vi "BotPose Correction.vi"(9 "Pos In":cluster{"x":dbl, "y":dbl}={"x"=13.014915967536774, "y"=9.532980345268305}, 10 "Robot Velocities In":T3={"X Velocity"=-6.0927338461737115e-19, "Y Velocity"=3.330663501205842e-16, "Rotational \nVelocity"=-0.0823974609375}) -> (0 "BotPose":cluster{"Numeric":dbl, "Numeric":dbl}, 1 "Bordeaux Pos":cluster{dbl, dbl}, 2 "Robot Velocities Out":T3={"X Velocity"=-6.0927338461737115e-19, "Y Velocity"=3.330663501205842e-16, "Rotational \nVelocity"=-0.0823974609375})   [LabVIEW 2025]
uses:
  swerve-template/Type Definitions/Data/Robot Velocities.ctl
  <vilib>/Rock Robotics/Network Tables/NT Read Numeric Array.vi
  <vilib>/addons/control/pid/pid.llb/PID (DBL).vi
  <vilib>/addons/control/pid/NI_PID_pid.lvlib
panel:
  in  "PID gains":T1={"proportional gain (Kc)"=2.5, "integral time (Ti, min)"=0.0, "derivative time (Td, min)"=0.0} {"derivative time (Td, min)" format="%.3f"; "integral time (Ti, min)" format="%.3f"; "proportional gain (Kc)" format="%.3f"}
  in  "output range":cluster{"output high":dbl, "output low":dbl}={"output high"=4.0, "output low"=-4.0} {"output low" format="%.2f"; "output high" format="%.2f"}
  out "Error":cluster{dbl, dbl}(graph)={-6.0927338461737115e-19, -1.21152228156357}
  out "Velocities OUT":T2(graph)={"X Velocity"=-6.0927338461737115e-19, "Y Velocity"=3.330663501205842e-16, "Rotational \nVelocity"=-0.0823974609375}
  out "Tag IDs":dbl(graph)=18.0
  out "Correction":cluster{dbl, dbl}(graph)={-6.0927338461737115e-19, -1.21152228156357}
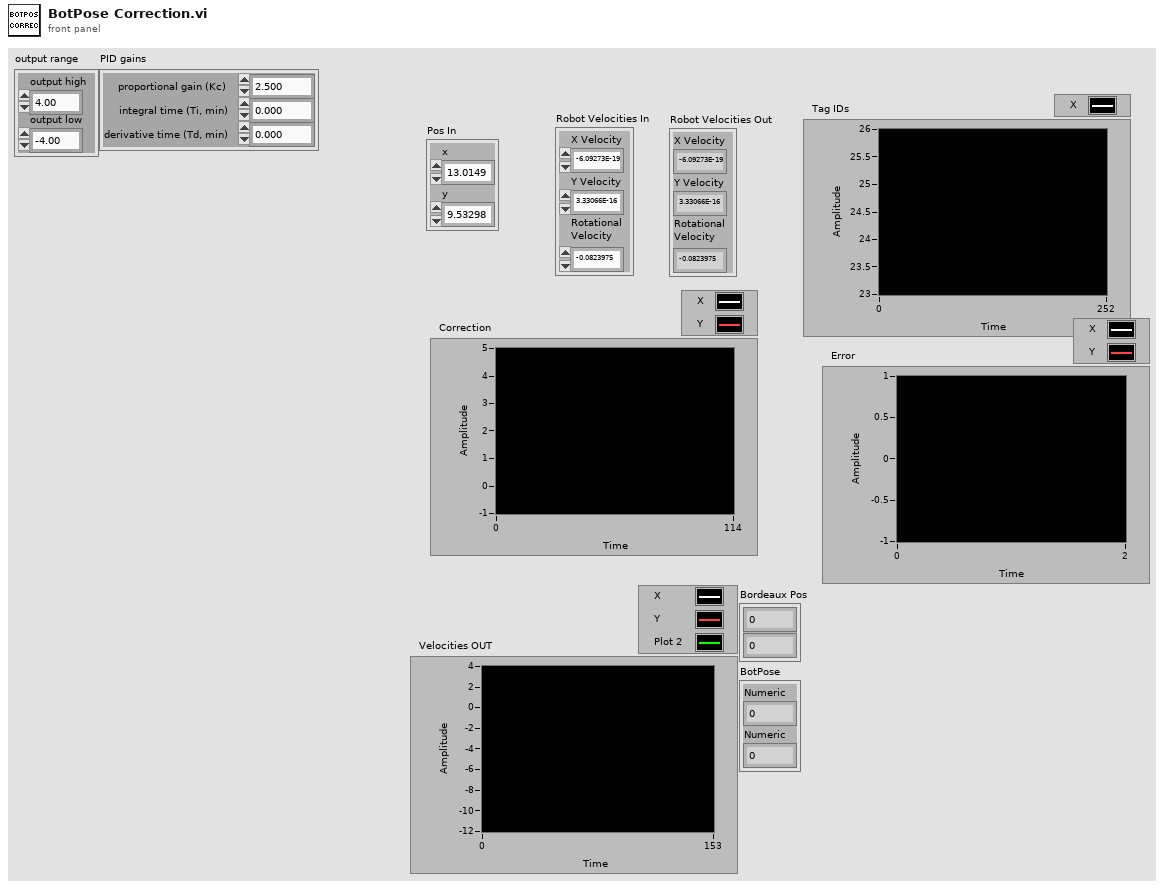
[diagram p1: front panel]
types:
  T1 = cluster{"proportional gain (Kc)":dbl, "integral time (Ti, min)":dbl, "derivative time (Td, min)":dbl}
  T2 = cluster{"X Velocity":dbl, "Y Velocity":dbl, "Rotational \nVelocity":dbl}
  T3 = typedef "Robot Velocities.ctl" = cluster{"X Velocity":dbl, "Y Velocity":dbl, "Rotational \nVelocity":dbl}
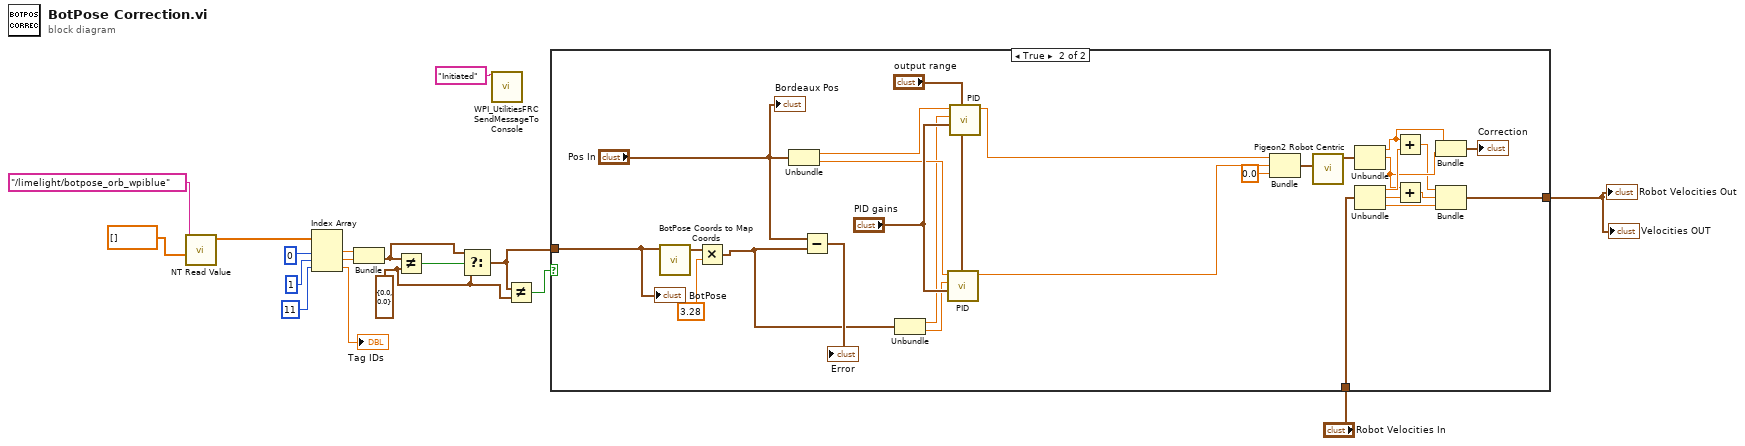
[diagram p0: block diagram]
diagram:
  w1 = cluster{"Numeric":dbl, "Numeric":dbl} {"Numeric"=0.0, "Numeric"=0.0} ("y")
  n1 = call-poly <vilib>:"NT Read Value.vi"("default value"=dbl[] [], "name"="/limelight/botpose_orb_wpiblue") -> ("value"=w16:dbl[])  [unwired: 7 in, 2 out]
  n2 = Index Array(array=w16, index #1=0 ("index"), index #2=1 ("index"), index #3=11 ("index")) -> (element #1=w7:dbl, element #2=w6:dbl, element #3=→"Tag IDs":dbl)
  n3 = Bundle("Numeric"=w7, "Numeric"=w6) -> (w4:cluster{"Numeric":dbl, "Numeric":dbl})  [unwired: 1 in]
  n4 = Not Equal?(x=w4, y=w1) -> (x != y?=w5:bool)
  n5 = Select(t=w4, s=w5, f=w1) -> (s? t:f=w2:cluster{"Numeric":dbl, "Numeric":dbl})
  n6 = call <vilib>:"WPI_UtilitiesFRC SendMessageToConsole.vi"("Message"="Initiated") -> ()  [unwired: 14 in, 1 out]
  n7 = Not Equal?(x=w2, y=w1) -> (x != y?=w3:bool)
  n8 = case shown="True" w3 {
    tunnel: w2 -> [_ w22]
    tunnel: [w18 w33] -> w10
    tunnel: "Robot Velocities In" -> [w18 w45]
    frame False {
    }
    frame True {
      n9 = call "BotPose Coords to Map Coords.vi"("Point In"=w22) -> ("Point Out"=w21:cluster{dbl, dbl})  [unwired: 10 in]
      n10 = Multiply(x=w21, y=3.28) -> (x*y=w19:cluster{dbl, dbl})
      n11 = Unbundle("Pos In") -> ("x"=w29:dbl, "y"=w28:dbl)
      n12 = Subtract(x="Pos In", y=w19) -> (x-y=→"Error":cluster{dbl, dbl})
      n13 = Unbundle(w19) -> (w27:dbl, w26:dbl)
      n14 = call-poly <vilib>:"PID.vi"("output range"="output range", "PID gains"="PID gains", "process variable"=w26, "setpoint"=w28) -> ("output"=w24:dbl)  [unwired: 6 in, 1 out]
      n15 = call-poly <vilib>:"PID.vi"("output range"="output range", "PID gains"="PID gains", "process variable"=w27, "setpoint"=w29) -> ("output"=w25:dbl)  [unwired: 6 in, 1 out]
      n16 = Bundle("output"=w25, "output"=w24, 0.0) -> (w42:cluster{"output":dbl, "output":dbl, dbl})  [unwired: 1 in]
      n17 = call "Pigeon2 Robot Centric.vi"("Robot Centric Velocities"=w42) -> ("Field Centric Velocities"=w41:T3)  [unwired: 10 in]
      n18 = Unbundle(w41) -> ("X Velocity"=w35:dbl, "Y Velocity"=w34:dbl)  [unwired: 1 out]
      n19 = Unbundle(w45) -> ("X Velocity"=w36:dbl, "Y Velocity"=w39:dbl, "Rotational \nVelocity"=w43:dbl)
      n20 = Add(x=w35, y=w36) -> (x+y=w32:dbl)
      n21 = Add(x=w34, y=w39) -> (x+y=w38:dbl)
      n22 = Bundle("X Velocity"=w35, "Y Velocity"=w34) -> (→"Correction":cluster{"X Velocity":dbl, "Y Velocity":dbl})  [unwired: 1 in]
      n23 = Bundle(w32, w38, "Rotational \nVelocity"=w43) -> (w33:cluster{dbl, dbl, "Rotational \nVelocity":dbl})  [unwired: 1 in]
      "Bordeaux Pos" <- "Pos In"
      "BotPose" <- w22
    }
  }
  "Robot Velocities Out" <- w10
  "Velocities OUT" <- w10
